vi "LINX - Set RGB LED Color.vi"() -> ()   [LabVIEW 2020]
doc: "Set the color of an RGB LED using three PWM channels."
uses:
  vi.lib/MakerHub/LINX/LMH-LINX.lvlib
  vi.lib/MakerHub/LINX/Public/Utilities/Open Serial.vi
  vi.lib/MakerHub/LINX/Private/Device/Device.lvlib
panel:
  in  "Blue PWM Channel":u8=6
  in  "Green PWM Channel":u8=5
  in  "Red PWM Channel":u8=3
  out "LED Color":u32(colorbox)
  in  "Blue":u8(slide) scale=0.0..255.0
  in  "Green":u8(slide) scale=0.0..255.0
  in  "Red":u8(slide) scale=0.0..255.0
  out "Loop Rate (Hz)":u32
  in  "Serial Port":refnum<visa-resource-name>
  in  "Stop Button":bool
  # "Circuit Schematic"
  # "LINX Device Settings"
  # "RGB LED Color"
  # "RGB LED Example\n\nThis example demonstrates how to set the color of an RGB LED using 3 PWM channels.\n\nNote: This example is configured to use a serial interface but can easily be modified\nto use TCP or run on myRIO.\n\nInstructions\n1. Select the COM Port associated with the LINX Device.\n2. Select the PWM Channels corresponding to the Red, Green, and Blue  LED leads.\n3. Click the Run Arrow.\n4. Adjust the Red, Green, and Blue sliders to change the BlinkM color."
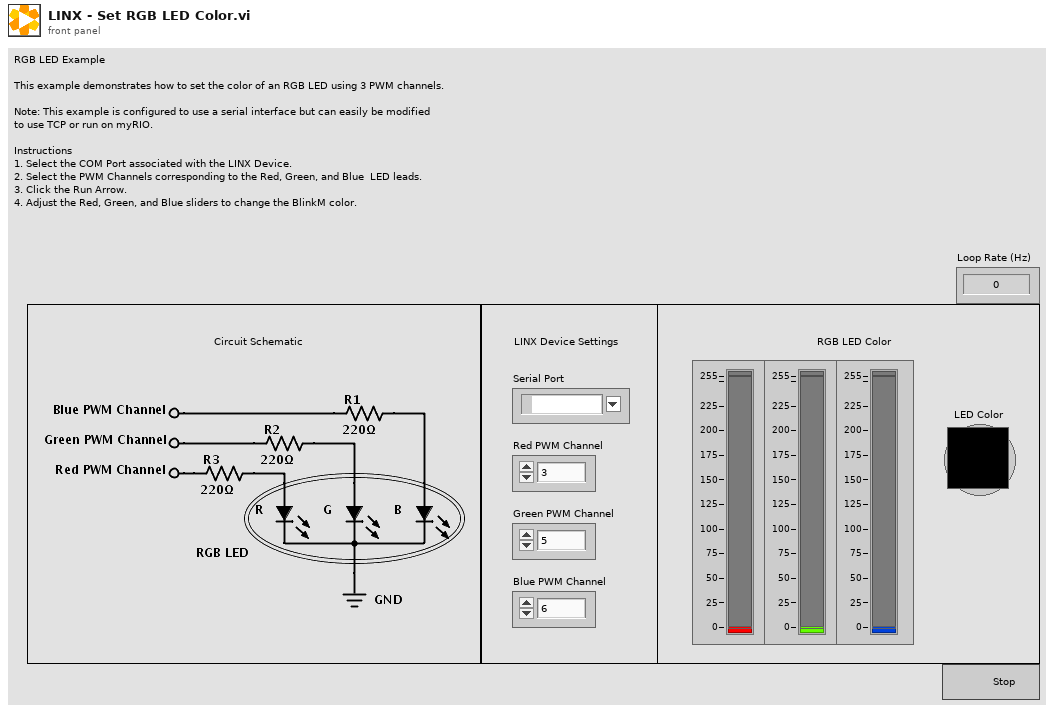
[diagram p1: front panel]
types:
  T1 = typedef "LMH-LINX.lvlib/LINX Ref.ctl" = cluster{"IO":T2, "Interface":T3, "LINX Device Config":T4}
  T2 = typedef "LMH-LINX.lvlib/Platform.ctl" = enum16{"Remote", "Local"}
  T3 = typedef "LMH-LINX.lvlib/Interface.ctl" = enum16{"Serial", "TCP"}
  T4 = typedef "Device.lvlib/LINX Device Config.ctl" = cluster{"Interface":T3, "COM Port":refnum<visa-resource-name>, "TCP Configuration":T5, "Device Family":u8, "Device ID":u8, "Device Name":string, "TCP Ref":refnum<k5>, "Channels":T6}
  T5 = typedef "Device.lvlib/TCP Config.ctl" = cluster{"IP Address":string, "Port":u16}
  T6 = typedef "LMH-LINX.lvlib/Channels.ctl" = cluster{"DI":u8[], "DO":u8[], "AI":u8[], "AO":u8[], "PWM":u8[], "QE":u8[], "UART":u8[], "I2C 2":u8[], "SPI":u8[], "CAN":u8[], "Servo":u8[], "AI Ref (V)":dbl, "AI Resolution (Bits)":u8, "AO Ref (V)":dbl, "AO Resolution (Bits)":u8}
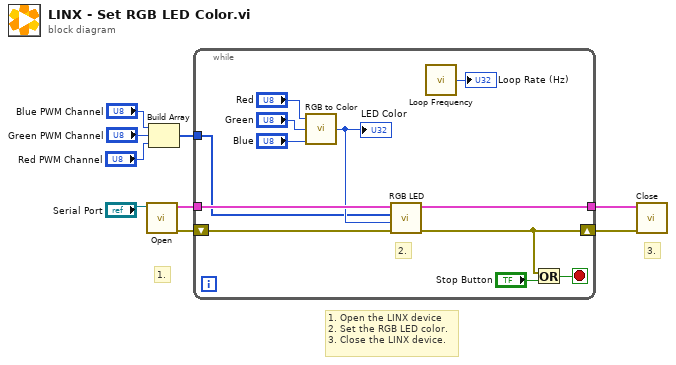
[diagram p0: block diagram]
diagram:
  # "3."
  # "1."
  # "1. Open the LINX device\n2. Set the RGB LED color.\n3. Close the LINX device."
  n1 = call-poly "Open.vi"("Serial Port"="Serial Port") -> ("Error Out"=w5:errorcluster, "LINX Resource"=w6:T1)  [unwired: 8 in, 1 out]
  n2 = Build Array("Blue PWM Channel", "Green PWM Channel", "Red PWM Channel") -> (w1:u8[])
  n3 = while {
    shift-right: [w18] -> w9
    shift-left: w5 -> [w17]
    tunnel: [w16] -> w7
    tunnel: w6 -> [w15]
    tunnel: w1 -> [w10]
    stop <- w21 stop-if-true
    # "2."
    n4 = call <vilib>:"RGB to Color.vi"("B"="Blue", "G"="Green", "R"="Red") -> ("Color"=w11:u32)
    "LED Color" <- w11
    n5 = call "RGB LED.vi"("Error In"=w17, "Color"=w11, "Channels (R, G, B)"=w10, "LINX Resource"=w15) -> ("Error Out"=w18:errorcluster, "LINX Resource"=w16:T1)  [unwired: 6 in]
    n6 = call "Loop Frequency.vi"() -> ("Loop Rate (Hz)"=→"Loop Rate (Hz)":u32)
    n7 = Or(x=w18, y="Stop Button") -> (x .or. y?=w21:bool)
  }
  n8 = call "Close.vi"("Error In"=w9, "LINX Resource"=w7) -> ()  [unwired: 9 in, 1 out]
